vi "Power (N Channels).vi"(8 "error in (no error)":errorcluster, 10 "current waveforms":waveform(dbl)[](array[waveform]), 11 "voltage waveforms":waveform(dbl)[](array[waveform])) -> (0 "error out":errorcluster, 3 "power values":T1[](array[typedef]))   [LabVIEW 2013, in "NI_EP_Basic.lvlib"]
doc: "Calculates the power values from a voltage and current signal. Wire data to the <B>voltage waveform</B> input or the <B>current waveform</B> input to determine the polymorphic instance to use or manually select the instance."
uses:
  <vilib>/addons/Electrical Power/Basic/NI_EP_Basic.lvlib
  <vilib>/addons/Electrical Power/Basic/Measurement/subVIs/basic_Power Value.ctl
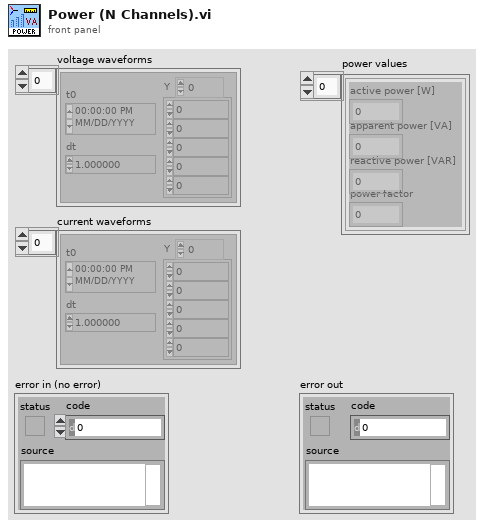
[diagram p1: front panel]
types:
  T1 = typedef "NI_EP_Basic.lvlib/basic_Power Value.ctl" = cluster{"active power [W]":dbl, "apparent power [VA]":dbl, "reactive power [VAR]":dbl, "power factor":dbl}
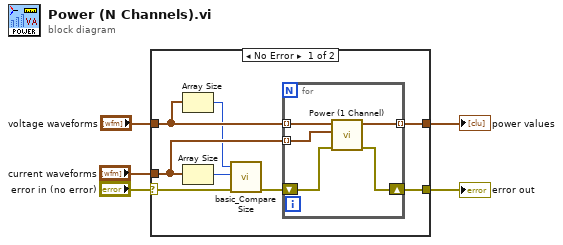
[diagram p0: block diagram]
diagram:
  n1 = case shown="No Error" "error in (no error)" {
    selector: "error in (no error)" -> [w8 w19]
    tunnel: "voltage waveforms" -> [w11 _]
    tunnel: "current waveforms" -> [w10 _]
    tunnel: [w13 w19] -> w2
    tunnel: [w12 _] -> w1
    frame No Error {
      n2 = Array Size(array=w11) -> (size(s)=w6:i32)
      n3 = Array Size(array=w10) -> (size(s)=w7:i32)
      n4 = call <vilib>:"basic_Compare Size.vi"("error in (no error)"=w8, "size B"=w7, "size A"=w6) -> ("error out"=w9:errorcluster)  [unwired: 8 in]
      n5 = for {
        tunnel: w11 -> [w18] mode=indexing
        tunnel: w10 -> [w17] mode=indexing
        shift-right: [w15] -> w13
        shift-left: w9 -> [w16]
        tunnel: [w14] -> w12 mode=indexing
        n6 = call <vilib>:"Power (1 Channel).vi"("error in (no error)"=w16, "current waveform"=w17, "voltage waveform"=w18) -> ("error out"=w15:errorcluster, "power value"=w14:T1)  [unwired: 7 in]
      }
    }
    frame Error {
    }
  }
  "error out" <- w2
  "power values" <- w1
